vi "TTS_MCC.vi"(4 "Volume":i32(slide)=100 min=0 max=100 scale=0.0..100.0, 5 "Rate":i32(slide) min=-10 max=10 scale=-10.0..10.0, 6 "Output Device":u16(ring) items=["Lautsprecher / Kopfhörer (IDT High Definition Audio CODEC)"], 7 "reference (Eingang)":refnum<vi>, 9 "Lisa":string, 10 "TTS Voice":u16(ring) items=["Microsoft Anna - English (United States)"], 11 "Ring (Eingang)":refnum<vi>) -> (3 "Speaking...":bool)   [LabVIEW 2021]
uses:
  String Changed__OGPI.vi
  SAPI_Speak_Text_String_SubVI.vi
  Users/sacha/Desktop/labview/TTS new 2012/SAPI TTS Library/SAPI.TTS.lvlib
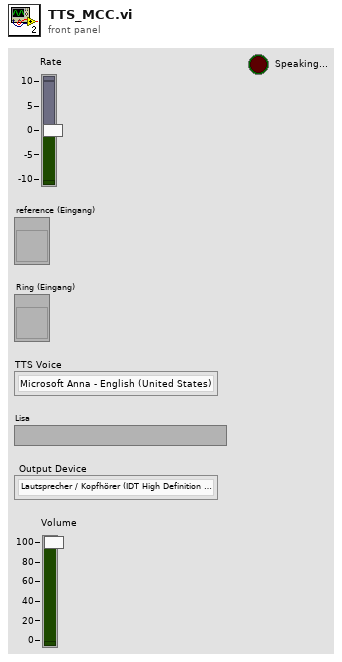
[diagram p1: front panel]
types:
  T1 = typedef "SAPI.TTS.lvlib/Speech object references.ctl" = cluster{"SpeechLib.ISpeechVoice":refnum<k7>, "GetVoices":refnum<k7>, "GetAudioOutputs":refnum<k7>}
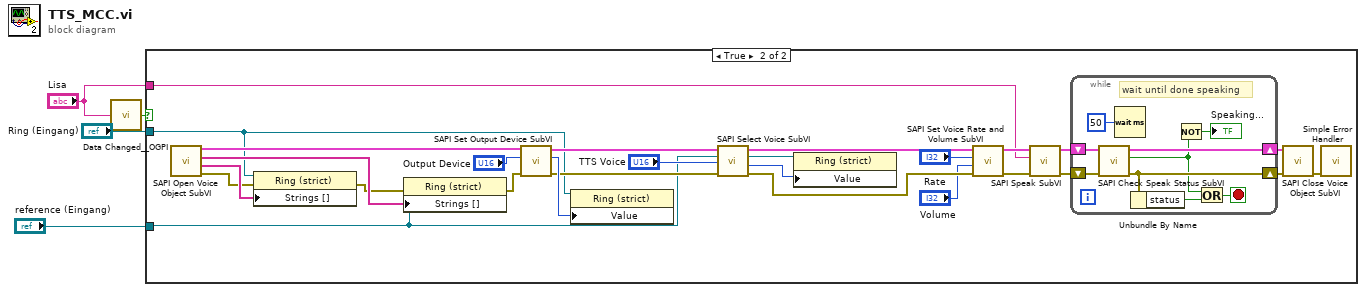
[diagram p0: block diagram]
diagram:
  n1 = call-poly "Data Changed__OGPI.vi"("String"="Lisa") -> ("Changed"=w4:bool)
  n2 = case shown="True" w4 {
    tunnel: "Lisa" -> [_ w7]
    tunnel: "Ring (Eingang)" -> [_ w6]
    tunnel: "reference (Eingang)" -> [_ w5]
    frame False {
    }
    frame True {
      n3 = call "SAPI Open Voice Object SubVI.vi"() -> ("error out"=w20:errorcluster, "AudioOutputs"=w21:string[], "Voice Names"=w15:string[], "speech object references"=w19:T1)  [unwired: 8 in]
      n4 = property on="Eigenschaftsknoten" class="Ring (strict)"(reference=w6, error in=w20, "Strings []"=w21) -> (error out=w12:errorcluster)  [unwired: 1 out]
      n5 = property on="Eigenschaftsknoten" class="Ring (strict)"(reference=w5, error in=w12, "Strings []"=w15) -> (error out=w11:errorcluster)  [unwired: 1 out]
      n6 = call "SAPI Set Output Device SubVI.vi"("error in (no error)"=w11, "Device Number"="Output Device", "speech object references"=w19) -> ("error out"=w10:errorcluster, "Device Number"=w16:u16, "speech object references (out)"=w18:T1)  [unwired: 6 in]
      n7 = property class="Ring (strict)"(reference=w6, "Value"=w16) -> ()  [unwired: 1 in, 2 out]
      n8 = call "SAPI Select Voice SubVI.vi"("error in (no error)"=w10, "Voice Index (default voice: 0)"="TTS Voice", "speech object references"=w18) -> ("error out"=w25:errorcluster, "Voice Index (coerced)"=w13:u16, "speech object references (out)"=w27:T1)  [unwired: 6 in]
      n9 = property class="Ring (strict)"(reference=w5, "Value"=w13) -> ()  [unwired: 1 in, 2 out]
      n10 = call "SAPI Set Voice Rate and Volume SubVI.vi"("error in (no error)"=w25, "Volume (0 to 100: 100)"="Volume", "Speech Rate (-10 to 10: 0)"="Rate", "speech object references"=w27) -> ("error out"=w24:errorcluster, "speech object references (out)"=w26:T1)  [unwired: 6 in]
      n11 = call-poly "SAPI Speak SubVI.vi"("error in (no error)"=w24, "Text to speak"=w7, "speech object references"=w26) -> ("error out"=w29:errorcluster, "speech object references (out)"=w30:T1)  [unwired: 7 in]
      n12 = while {
        shift-right: [w34] -> w8
        shift-left: w29 -> [w38]
        shift-right: [w35] -> w9
        shift-left: w30 -> [w39]
        stop <- w36 stop-if-true
        # "wait until done speaking"
        n13 = call "SAPI Check Speak Status SubVI.vi"("error in (no error)"=w38, "speech object references"=w39) -> ("error out"=w34:errorcluster, "Status (T: Done)"=w33:bool, "speech object references (out)"=w35:T1)  [unwired: 7 in]
        n14 = Wait (ms)(milliseconds to wait=u32 50) -> ()  [unwired: 1 out]
        n15 = Unbundle By Name(w34) -> ("status"=w37:bool)
        n16 = Not(x=w33) -> (.not. x?=→"Speaking...":bool)
        n17 = Or(x=w33, y=w37) -> (x .or. y?=w36:bool)
      }
      n18 = call "SAPI Close Voice Object SubVI.vi"("error in (no error)"=w8, "speech object references"=w9) -> ("error out"=w28:errorcluster)  [unwired: 9 in]
      n19 = call <vilib>:"Simple Error Handler.vi"("error in (no error)"=w28) -> ()  [unwired: 4 in, 5 out]
    }
  }
